vi "Flash DTM Mode.vi"(8 "error in":errorcluster, 10 "Hex File Name":string="direct_test_mode_pca10040.hex", 11 "nRF52 Serial Number (posted on the DUT)":string="1050336144") -> (0 "error out":errorcluster, 2 "standard error":string, 3 "standard output":string)   [LabVIEW 2026, in "Nordic nRF52 DK DTM Test.lvlib"]
uses:
  Nordic nRF52 DK DTM Test.lvlib
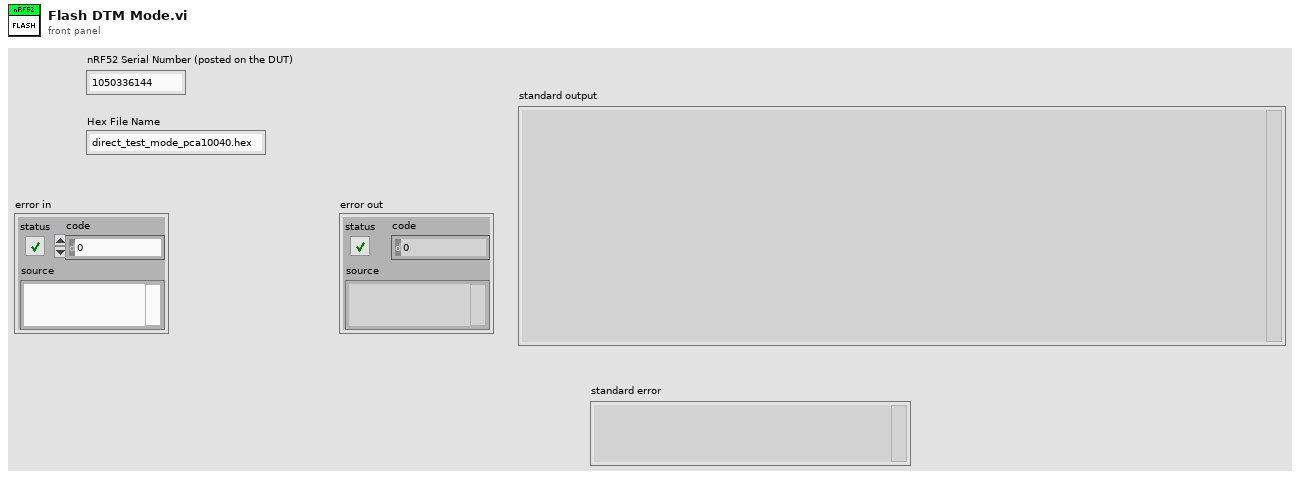
[diagram p1: front panel]
types:
  T1 = enum16{"open", "replace", "create", "open or create", "replace or create", "replace or create with confirmation"}
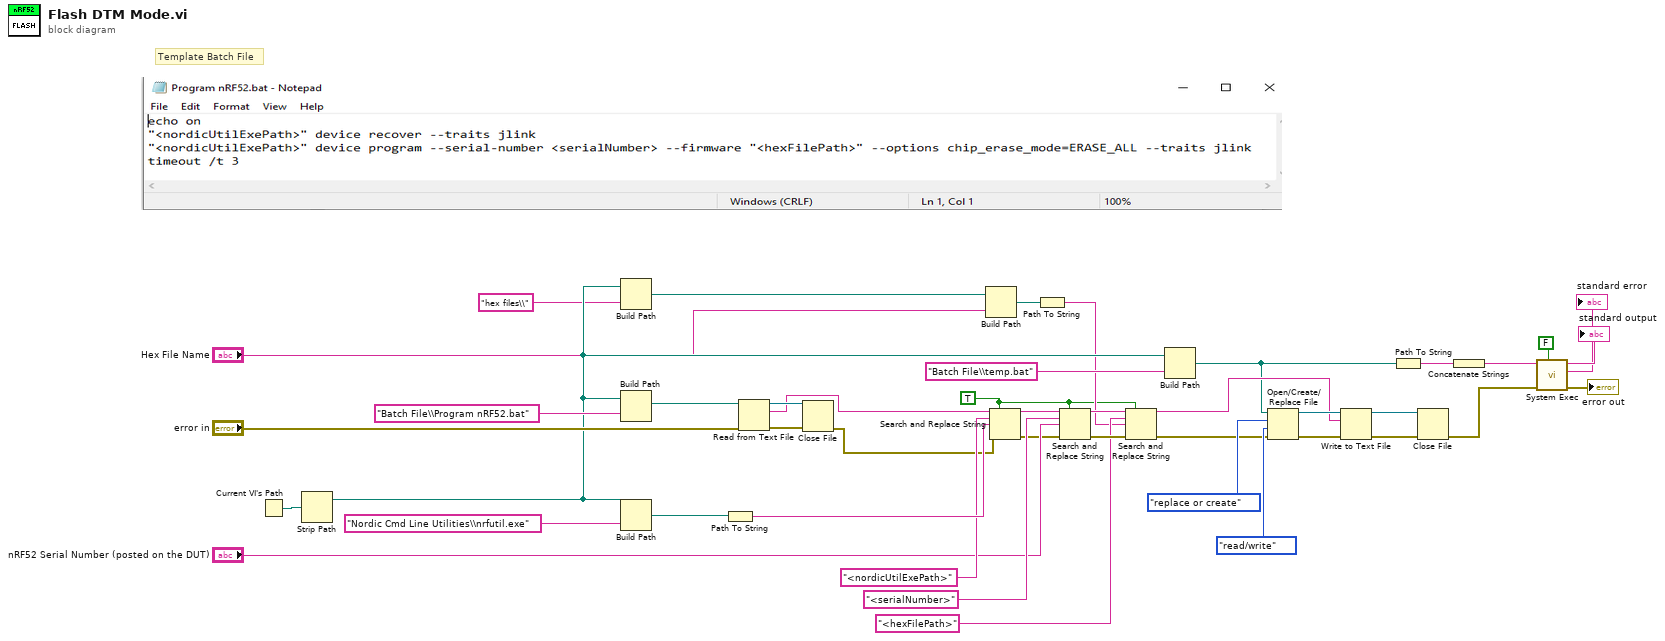
[diagram p0: block diagram]
diagram:
  w8 = TRUE ("replace all? (F)")
  # "Template Batch File"
  n1 = Current VI's Path() -> (path=w42:path)
  n2 = Strip Path(path=w42) -> (stripped path=w14:path)  [unwired: 1 out]
  n3 = Build Path(base path=w14, name or relative path="hex files\\" ("text")) -> (appended path=w12:path)
  n4 = Build Path(base path=w14, name or relative path="Batch File\\Program nRF52.bat" ("text")) -> (appended path=w41:path)
  n5 = Build Path(base path=w14, name or relative path="Nordic Cmd Line Utilities\\nrfutil.exe") -> (appended path=w39:path)
  n6 = Path To String(path=w39) -> (string=w38:string)
  n7 = Read from Text File(file (use dialog)=w41, error in="error in") -> (refnum out=w31:refnum<file>, text=w22:string, error out=w30:errorcluster)  [unwired: 2 in, 1 out]
  n8 = Close File(refnum=w31, error in=w30) -> (error out=w21:errorcluster)  [unwired: 1 out]
  n9 = Build Path(base path=w12, name or relative path="Hex File Name") -> (appended path=w10:path)
  n10 = Search and Replace String(replace all?=w8, input string=w22, search string="<nordicUtilExePath>", replace string=w38, error in=w21) -> (result string=w36:string, error out=w32:errorcluster)  [unwired: 3 in, 2 out]
  n11 = Path To String(path=w10) -> (string=w9:string)
  n12 = Search and Replace String(replace all?=w8, input string=w36, search string="<serialNumber>", replace string="nRF52 Serial Number (posted on the DUT)", error in=w32) -> (result string=w16:string, error out=w17:errorcluster)  [unwired: 3 in, 2 out]
  n13 = Search and Replace String(replace all?=w8, input string=w16, search string="<hexFilePath>", replace string=w9, error in=w17) -> (result string=w6:string, error out=w7:errorcluster)  [unwired: 3 in, 2 out]
  n14 = Build Path(base path=w14, name or relative path="Batch File\\temp.bat" ("text")) -> (appended path=w5:path)
  n15 = Open/Create/Replace File(file path (use dialog)=w5, error in=w7, operation (0:open)=T1."replace or create", access (0:read/write)=enum16{"read/write", "read-only", "write-only"}."read/write") -> (refnum out=w25:refnum<file>, error out=w28:errorcluster)  [unwired: 2 in, 1 out]
  n16 = Write to Text File(file (use dialog)=w25, text=w6, error in=w28) -> (refnum out=w23:refnum<file>, error out=w24:errorcluster)  [unwired: 1 in, 1 out]
  n17 = Path To String(path=w5) -> (string=w20:string)
  n18 = Close File(refnum=w23, error in=w24) -> (error out=w19:errorcluster)  [unwired: 1 out]
  n19 = Concatenate Strings(w20) -> (w18:string)
  n20 = call <vilib>:"System Exec.vi"("wait until completion? (T)"=FALSE, "error in (no error)"=w19, "command line"=w18) -> ("error out"=→"error out":errorcluster, "standard error"=→"standard error":string, "standard output"=→"standard output":string)  [unwired: 5 in, 1 out]
